vi "test.1dArrays.vi"(8 "error in":errorcluster, 10 "Data":variant, 11 "Command":string) -> (0 "error out":errorcluster, 3 "Return Data":variant)   [LabVIEW 2014]
uses:
  Private/Class/meth.Constructor.vi
  Private/Class/meth.Destructor.vi
  GLue.lvlib
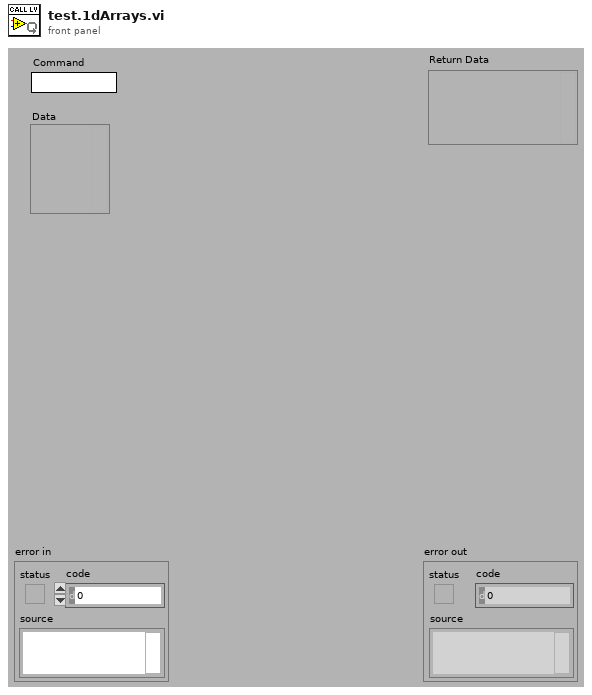
[diagram p1: front panel]
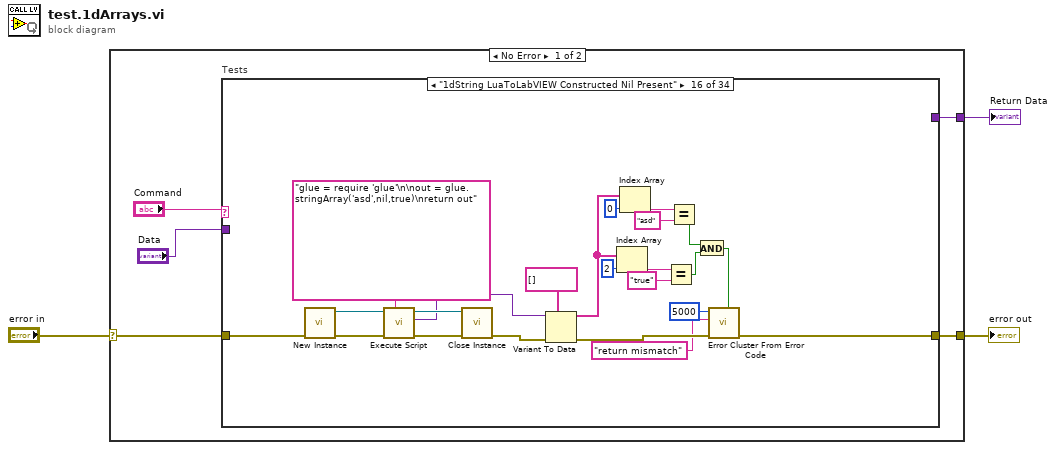
[diagram p0: block diagram]
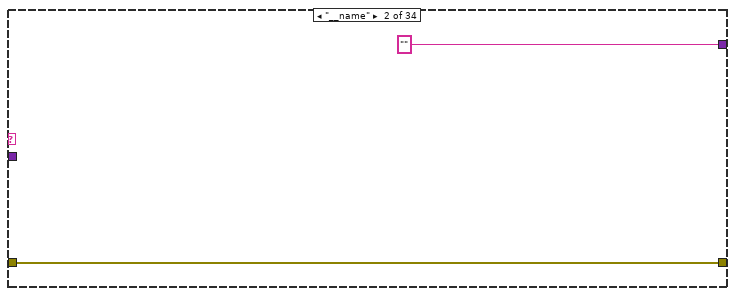
[diagram p3: hidden frame]
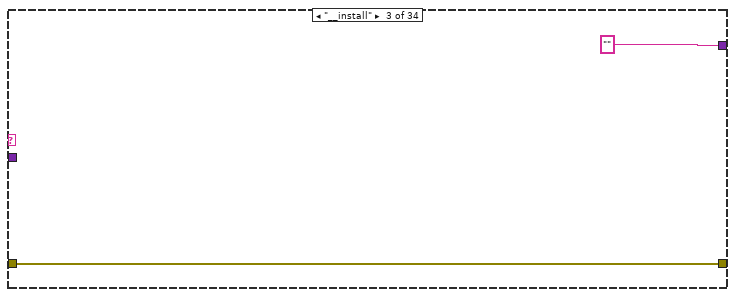
[diagram p4: hidden frame]
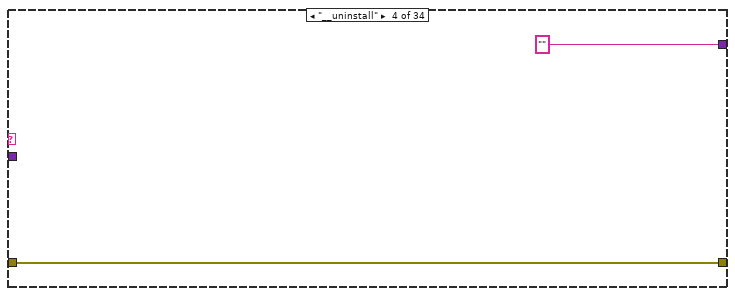
[diagram p5: hidden frame]
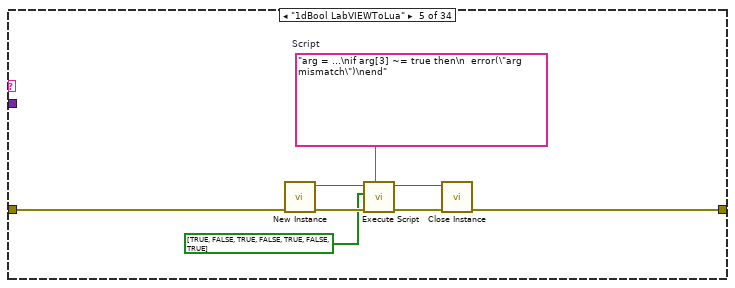
[diagram p6: hidden frame]
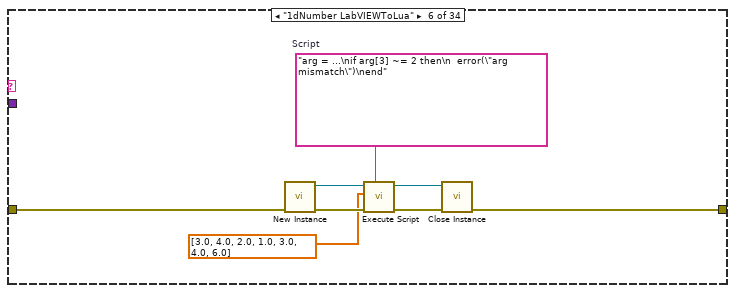
[diagram p7: hidden frame]
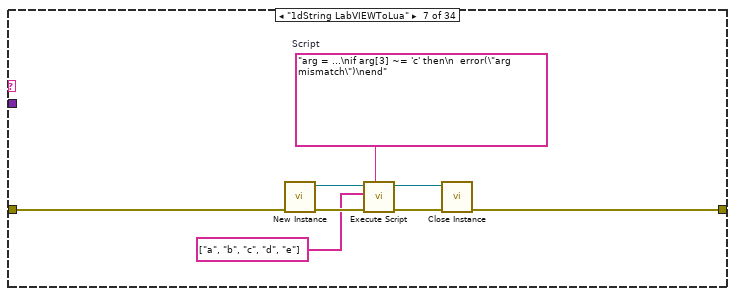
[diagram p8: hidden frame]
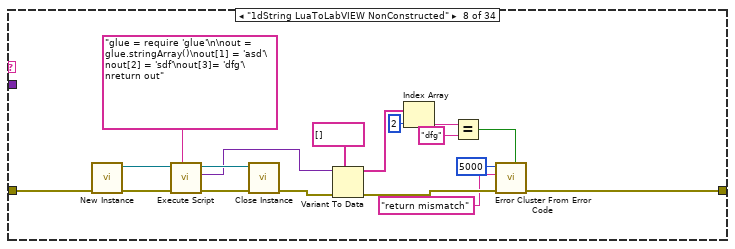
[diagram p9: hidden frame]
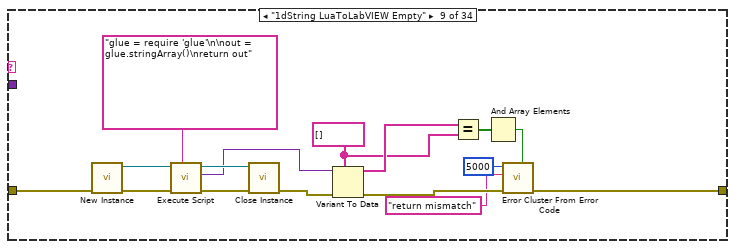
[diagram p10: hidden frame]
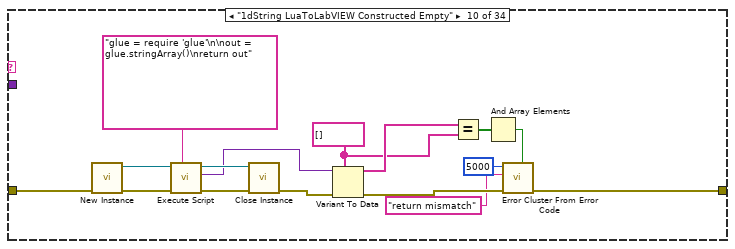
[diagram p11: hidden frame]
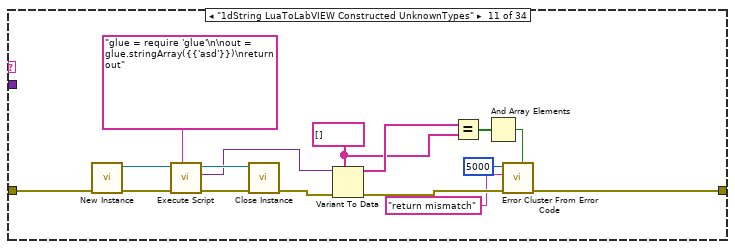
[diagram p12: hidden frame]
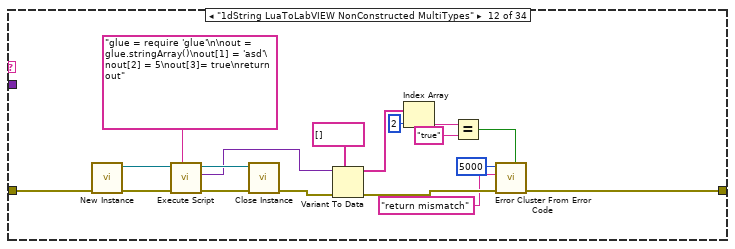
[diagram p13: hidden frame]
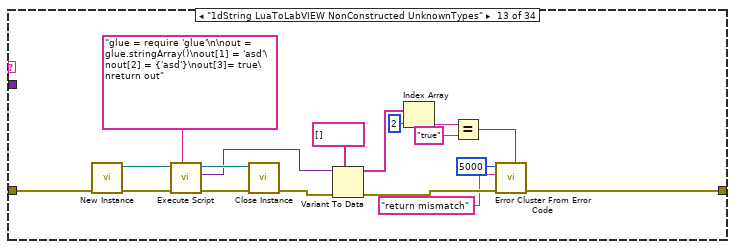
[diagram p14: hidden frame]
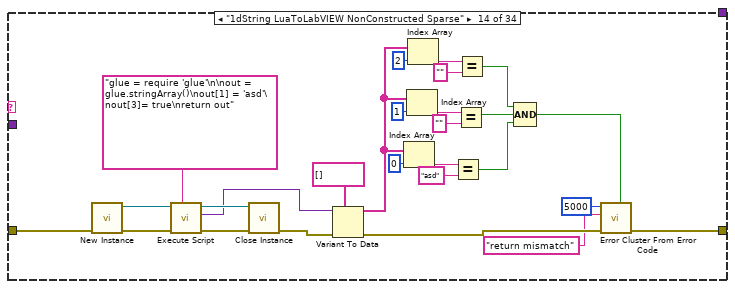
[diagram p15: hidden frame]
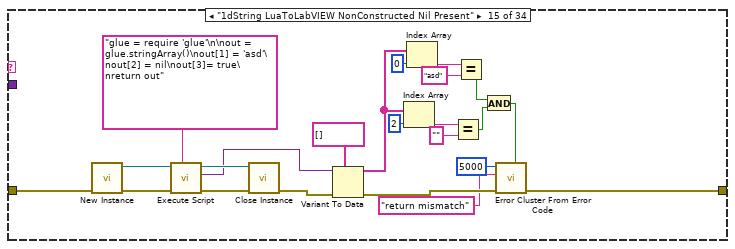
[diagram p16: hidden frame]
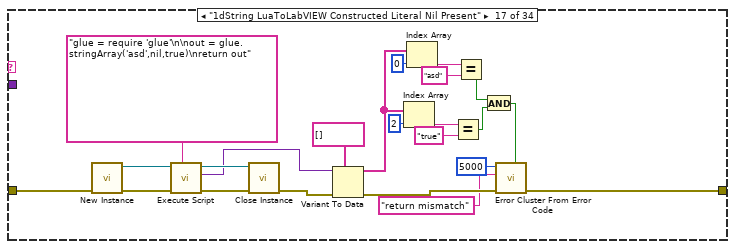
[diagram p17: hidden frame]
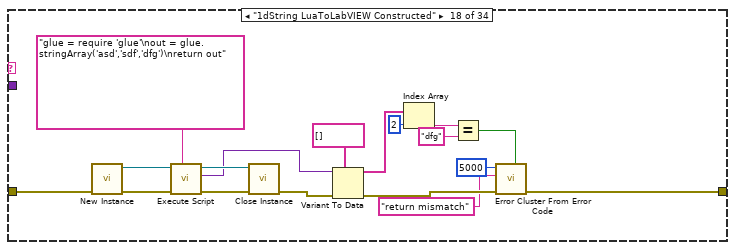
[diagram p18: hidden frame]
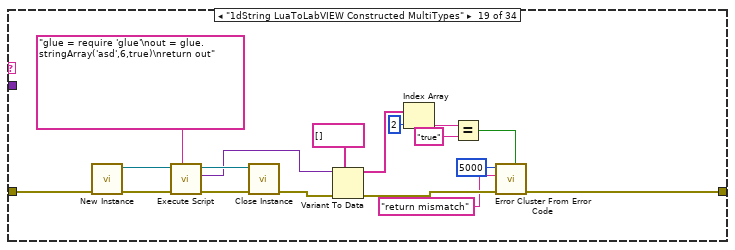
[diagram p19: hidden frame]
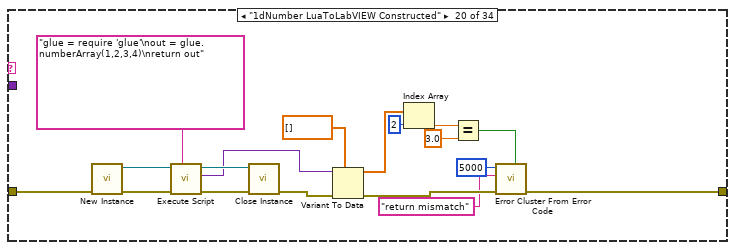
[diagram p20: hidden frame]
diagram:
  n1 = case shown="No Error" "error in" {
    selector: "error in" -> [w8 w579]
    tunnel: [w6 w579] -> w2
    tunnel: [w7 variant ("User Data")] -> w1
    frame No Error {
      n2 = case "Tests" shown="\"1dString LuaToLabVIEW Constructed Nil Present\"" "Command" {
        tunnel: w8 -> [w10 w11 w13 w15 w19 w27 w35 w53 w69 w85 w101 w119 w137 w164 w187 w210 w233 w251 w269 w287 w305 w321 w348 w375 w398 w420 w442 w459 w476 w494 w510 w526 w549 w572]
        tunnel: "Data" -> [w9 _ _ _ _ _ _ _ _ _ _ _ _ _ _ _ _ _ _ _ _ _ _ _ _ _ _ _ _ _ _ _ _ _]
        tunnel: [w9 "" "" "" _ _ _ _ _ _ _ _ _ _ _ _ _ _ _ _ _ _ _ _ _ _ _ _ _ _ _ _ _ _] -> w7
        tunnel: [w10 w11 w13 w15 w18 w26 w34 w48 w65 w81 w97 w114 w132 w159 w182 w205 w228 w246 w264 w283 w301 w317 w344 w371 w394 w416 w438 w455 w472 w490 w506 w522 w545 w568] -> w6
        frame Default {
        }
        frame "__name" {
        }
        frame "__install" {
        }
        frame "__uninstall" {
        }
        frame "1dBool LabVIEWToLua" {
          w24 = "arg = ...\nif arg[3] ~= true then\n  error(\"arg mismatch\")\nend"  # Script
          n3 = call "New Instance.vi"("error in"=w19) -> ("error out"=w20:errorcluster, "GLue out"=w21:refnum<class "class.GLue.lvclass">)  [unwired: 9 in]
          n4 = call "Execute Script.vi"("Script"=w24, "error in"=w20, "Argument Data"=bool[] [TRUE, FALSE, TRUE, FALSE, TRUE, FALSE, TRUE], "GLue in"=w21) -> ("error out"=w22:errorcluster, "GLue out"=w23:refnum<class "class.GLue.lvclass">)  [unwired: 5 in, 1 out]
          n5 = call "Close Instance.vi"("error in"=w22, "GLue in"=w23) -> ("error out"=w18:errorcluster)  [unwired: 9 in]
        }
        frame "1dNumber LabVIEWToLua" {
          w32 = "arg = ...\nif arg[3] ~= 2 then\n  error(\"arg mismatch\")\nend"  # Script
          n6 = call "New Instance.vi"("error in"=w27) -> ("error out"=w28:errorcluster, "GLue out"=w29:refnum<class "class.GLue.lvclass">)  [unwired: 9 in]
          n7 = call "Execute Script.vi"("Script"=w32, "error in"=w28, "Argument Data"=dbl[] [3.0, 4.0, 2.0, 1.0, 3.0, 4.0, 6.0], "GLue in"=w29) -> ("error out"=w30:errorcluster, "GLue out"=w31:refnum<class "class.GLue.lvclass">)  [unwired: 5 in, 1 out]
          n8 = call "Close Instance.vi"("error in"=w30, "GLue in"=w31) -> ("error out"=w26:errorcluster)  [unwired: 9 in]
        }
        frame "1dString LabVIEWToLua" {
          w40 = "arg = ...\nif arg[3] ~= 'c' then\n  error(\"arg mismatch\")\nend"  # Script
          n9 = call "New Instance.vi"("error in"=w35) -> ("error out"=w36:errorcluster, "GLue out"=w37:refnum<class "class.GLue.lvclass">)  [unwired: 9 in]
          n10 = call "Execute Script.vi"("Script"=w40, "error in"=w36, "Argument Data"=string[] ["a", "b", "c", "d", "e"], "GLue in"=w37) -> ("error out"=w38:errorcluster, "GLue out"=w39:refnum<class "class.GLue.lvclass">)  [unwired: 5 in, 1 out]
          n11 = call "Close Instance.vi"("error in"=w38, "GLue in"=w39) -> ("error out"=w34:errorcluster)  [unwired: 9 in]
        }
        frame "1dString LuaToLabVIEW NonConstructed" {
          n12 = call "New Instance.vi"("error in"=w53) -> ("error out"=w54:errorcluster, "GLue out"=w55:refnum<class "class.GLue.lvclass">)  [unwired: 9 in]
          n13 = call "Execute Script.vi"("Script"="glue = require 'glue'\n\nout = glue.stringArray()\nout[1] = 'asd'\nout[2] = 'sdf'\nout[3]= 'dfg'\nreturn out", "error in"=w54, "GLue in"=w55) -> ("error out"=w56:errorcluster, "Return Data"=w51:variant, "GLue out"=w57:refnum<class "class.GLue.lvclass">)  [unwired: 6 in]
          n14 = call "Close Instance.vi"("error in"=w56, "GLue in"=w57) -> ("error out"=w52:errorcluster)  [unwired: 9 in]
          n15 = Variant To Data(error in=w52, type=string[] [], Variant=w51) -> (data=w47:string[], error out=w49:errorcluster)
          n16 = Index Array(array=w47, index=2) -> (element=w45:string)
          n17 = Equal?(x=w45, y="dfg") -> (x = y?=w43:bool)
          n18 = call <vilib>:"Error Cluster From Error Code.vi"("is warning? (False)"=w43, "error in (no error)"=w49, "error message (\"\")"="return mismatch" ("error message (\"\")"), "error code (0)"=5000) -> ("error out"=w48:errorcluster)  [unwired: 5 in]
        }
        frame "1dString LuaToLabVIEW Empty" {
          w61 = string[] []
          n19 = call "New Instance.vi"("error in"=w69) -> ("error out"=w70:errorcluster, "GLue out"=w71:refnum<class "class.GLue.lvclass">)  [unwired: 9 in]
          n20 = call "Execute Script.vi"("Script"="glue = require 'glue'\n\nout = glue.stringArray()\nreturn out", "error in"=w70, "GLue in"=w71) -> ("error out"=w72:errorcluster, "Return Data"=w67:variant, "GLue out"=w73:refnum<class "class.GLue.lvclass">)  [unwired: 6 in]
          n21 = call "Close Instance.vi"("error in"=w72, "GLue in"=w73) -> ("error out"=w68:errorcluster)  [unwired: 9 in]
          n22 = Variant To Data(error in=w68, type=w61, Variant=w67) -> (data=w62:string[], error out=w66:errorcluster)
          n23 = Equal?(x=w62, y=w61) -> (x = y?=w60:bool[])
          n24 = And Array Elements(Boolean array=w60) -> (logical AND=w59:bool)
          n25 = call <vilib>:"Error Cluster From Error Code.vi"("is warning? (False)"=w59, "error in (no error)"=w66, "error message (\"\")"="return mismatch" ("error message (\"\")"), "error code (0)"=5000) -> ("error out"=w65:errorcluster)  [unwired: 5 in]
        }
        frame "1dString LuaToLabVIEW Constructed Empty" {
          w77 = string[] []
          n26 = call "New Instance.vi"("error in"=w85) -> ("error out"=w86:errorcluster, "GLue out"=w87:refnum<class "class.GLue.lvclass">)  [unwired: 9 in]
          n27 = call "Execute Script.vi"("Script"="glue = require 'glue'\n\nout = glue.stringArray()\nreturn out", "error in"=w86, "GLue in"=w87) -> ("error out"=w88:errorcluster, "Return Data"=w83:variant, "GLue out"=w89:refnum<class "class.GLue.lvclass">)  [unwired: 6 in]
          n28 = call "Close Instance.vi"("error in"=w88, "GLue in"=w89) -> ("error out"=w84:errorcluster)  [unwired: 9 in]
          n29 = Variant To Data(error in=w84, type=w77, Variant=w83) -> (data=w78:string[], error out=w82:errorcluster)
          n30 = Equal?(x=w78, y=w77) -> (x = y?=w76:bool[])
          n31 = And Array Elements(Boolean array=w76) -> (logical AND=w75:bool)
          n32 = call <vilib>:"Error Cluster From Error Code.vi"("is warning? (False)"=w75, "error in (no error)"=w82, "error message (\"\")"="return mismatch" ("error message (\"\")"), "error code (0)"=5000) -> ("error out"=w81:errorcluster)  [unwired: 5 in]
        }
        frame "1dString LuaToLabVIEW Constructed UnknownTypes" {
          w93 = string[] []
          n33 = call "New Instance.vi"("error in"=w101) -> ("error out"=w102:errorcluster, "GLue out"=w103:refnum<class "class.GLue.lvclass">)  [unwired: 9 in]
          n34 = call "Execute Script.vi"("Script"="glue = require 'glue'\n\nout = glue.stringArray({{'asd'}})\nreturn out", "error in"=w102, "GLue in"=w103) -> ("error out"=w104:errorcluster, "Return Data"=w99:variant, "GLue out"=w105:refnum<class "class.GLue.lvclass">)  [unwired: 6 in]
          n35 = call "Close Instance.vi"("error in"=w104, "GLue in"=w105) -> ("error out"=w100:errorcluster)  [unwired: 9 in]
          n36 = Variant To Data(error in=w100, type=w93, Variant=w99) -> (data=w94:string[], error out=w98:errorcluster)
          n37 = Equal?(x=w94, y=w93) -> (x = y?=w92:bool[])
          n38 = And Array Elements(Boolean array=w92) -> (logical AND=w91:bool)
          n39 = call <vilib>:"Error Cluster From Error Code.vi"("is warning? (False)"=w91, "error in (no error)"=w98, "error message (\"\")"="return mismatch" ("error message (\"\")"), "error code (0)"=5000) -> ("error out"=w97:errorcluster)  [unwired: 5 in]
        }
        frame "1dString LuaToLabVIEW NonConstructed MultiTypes" {
          n40 = call "New Instance.vi"("error in"=w119) -> ("error out"=w120:errorcluster, "GLue out"=w121:refnum<class "class.GLue.lvclass">)  [unwired: 9 in]
          n41 = call "Execute Script.vi"("Script"="glue = require 'glue'\n\nout = glue.stringArray()\nout[1] = 'asd'\nout[2] = 5\nout[3]= true\nreturn out", "error in"=w120, "GLue in"=w121) -> ("error out"=w122:errorcluster, "Return Data"=w117:variant, "GLue out"=w123:refnum<class "class.GLue.lvclass">)  [unwired: 6 in]
          n42 = call "Close Instance.vi"("error in"=w122, "GLue in"=w123) -> ("error out"=w118:errorcluster)  [unwired: 9 in]
          n43 = Variant To Data(error in=w118, type=string[] [], Variant=w117) -> (data=w113:string[], error out=w115:errorcluster)
          n44 = Index Array(array=w113, index=2) -> (element=w111:string)
          n45 = Equal?(x=w111, y="true") -> (x = y?=w109:bool)
          n46 = call <vilib>:"Error Cluster From Error Code.vi"("is warning? (False)"=w109, "error in (no error)"=w115, "error message (\"\")"="return mismatch" ("error message (\"\")"), "error code (0)"=5000) -> ("error out"=w114:errorcluster)  [unwired: 5 in]
        }
        frame "1dString LuaToLabVIEW NonConstructed UnknownTypes" {
          n47 = call "New Instance.vi"("error in"=w137) -> ("error out"=w138:errorcluster, "GLue out"=w139:refnum<class "class.GLue.lvclass">)  [unwired: 9 in]
          n48 = call "Execute Script.vi"("Script"="glue = require 'glue'\n\nout = glue.stringArray()\nout[1] = 'asd'\nout[2] = {'asd'}\nout[3]= true\nreturn out", "error in"=w138, "GLue in"=w139) -> ("error out"=w140:errorcluster, "Return Data"=w135:variant, "GLue out"=w141:refnum<class "class.GLue.lvclass">)  [unwired: 6 in]
          n49 = call "Close Instance.vi"("error in"=w140, "GLue in"=w141) -> ("error out"=w136:errorcluster)  [unwired: 9 in]
          n50 = Variant To Data(error in=w136, type=string[] [], Variant=w135) -> (data=w131:string[], error out=w133:errorcluster)
          n51 = Index Array(array=w131, index=2) -> (element=w129:string)
          n52 = Equal?(x=w129, y="true") -> (x = y?=w127:bool)
          n53 = call <vilib>:"Error Cluster From Error Code.vi"("is warning? (False)"=w127, "error in (no error)"=w133, "error message (\"\")"="return mismatch" ("error message (\"\")"), "error code (0)"=5000) -> ("error out"=w132:errorcluster)  [unwired: 5 in]
        }
        frame "1dString LuaToLabVIEW NonConstructed Sparse" {
          n54 = call "New Instance.vi"("error in"=w164) -> ("error out"=w165:errorcluster, "GLue out"=w166:refnum<class "class.GLue.lvclass">)  [unwired: 9 in]
          n55 = call "Execute Script.vi"("Script"="glue = require 'glue'\n\nout = glue.stringArray()\nout[1] = 'asd'\nout[3]= true\nreturn out", "error in"=w165, "GLue in"=w166) -> ("error out"=w167:errorcluster, "Return Data"=w162:variant, "GLue out"=w168:refnum<class "class.GLue.lvclass">)  [unwired: 6 in]
          n56 = call "Close Instance.vi"("error in"=w167, "GLue in"=w168) -> ("error out"=w163:errorcluster)  [unwired: 9 in]
          n57 = Variant To Data(error in=w163, type=string[] [], Variant=w162) -> (data=w147:string[], error out=w160:errorcluster)
          n58 = Index Array(array=w147, index=0) -> (element=w157:string)
          n59 = Index Array(array=w147, index=1) -> (element=w152:string)
          n60 = Index Array(array=w147, index=2) -> (element=w149:string)
          n61 = Equal?(x=w157, y="asd") -> (x = y?=w144:bool)
          n62 = Equal?(x=w152, y="") -> (x = y?=w145:bool)
          n63 = Equal?(x=w149, y="") -> (x = y?=w146:bool)
          n64 = Compound Arithmetic op=AND(w146, w145, w144) -> (w143:bool)
          n65 = call <vilib>:"Error Cluster From Error Code.vi"("is warning? (False)"=w143, "error in (no error)"=w160, "error message (\"\")"="return mismatch" ("error message (\"\")"), "error code (0)"=5000) -> ("error out"=w159:errorcluster)  [unwired: 5 in]
        }
        frame "1dString LuaToLabVIEW NonConstructed Nil Present" {
          n66 = call "New Instance.vi"("error in"=w187) -> ("error out"=w188:errorcluster, "GLue out"=w189:refnum<class "class.GLue.lvclass">)  [unwired: 9 in]
          n67 = call "Execute Script.vi"("Script"="glue = require 'glue'\n\nout = glue.stringArray()\nout[1] = 'asd'\nout[2] = nil\nout[3]= true\nreturn out", "error in"=w188, "GLue in"=w189) -> ("error out"=w190:errorcluster, "Return Data"=w185:variant, "GLue out"=w191:refnum<class "class.GLue.lvclass">)  [unwired: 6 in]
          n68 = call "Close Instance.vi"("error in"=w190, "GLue in"=w191) -> ("error out"=w186:errorcluster)  [unwired: 9 in]
          n69 = Variant To Data(error in=w186, type=string[] [], Variant=w185) -> (data=w173:string[], error out=w183:errorcluster)
          n70 = Index Array(array=w173, index=2) -> (element=w180:string)
          n71 = Index Array(array=w173, index=0) -> (element=w175:string)
          n72 = Equal?(x=w180, y="") -> (x = y?=w171:bool)
          n73 = Equal?(x=w175, y="asd") -> (x = y?=w172:bool)
          n74 = And(x=w172, y=w171) -> (x .and. y?=w170:bool)
          n75 = call <vilib>:"Error Cluster From Error Code.vi"("is warning? (False)"=w170, "error in (no error)"=w183, "error message (\"\")"="return mismatch" ("error message (\"\")"), "error code (0)"=5000) -> ("error out"=w182:errorcluster)  [unwired: 5 in]
        }
        frame "1dString LuaToLabVIEW Constructed Nil Present" {
          n76 = call "New Instance.vi"("error in"=w210) -> ("error out"=w211:errorcluster, "GLue out"=w212:refnum<class "class.GLue.lvclass">)  [unwired: 9 in]
          n77 = call "Execute Script.vi"("Script"="glue = require 'glue'\n\nout = glue.stringArray('asd',nil,true)\nreturn out", "error in"=w211, "GLue in"=w212) -> ("error out"=w213:errorcluster, "Return Data"=w208:variant, "GLue out"=w214:refnum<class "class.GLue.lvclass">)  [unwired: 6 in]
          n78 = call "Close Instance.vi"("error in"=w213, "GLue in"=w214) -> ("error out"=w209:errorcluster)  [unwired: 9 in]
          n79 = Variant To Data(error in=w209, type=string[] [], Variant=w208) -> (data=w197:string[], error out=w206:errorcluster)
          n80 = Index Array(array=w197, index=2) -> (element=w203:string)
          n81 = Index Array(array=w197, index=0) -> (element=w199:string)
          n82 = Equal?(x=w203, y="true") -> (x = y?=w195:bool)
          n83 = Equal?(x=w199, y="asd") -> (x = y?=w196:bool)
          n84 = And(x=w196, y=w195) -> (x .and. y?=w194:bool)
          n85 = call <vilib>:"Error Cluster From Error Code.vi"("is warning? (False)"=w194, "error in (no error)"=w206, "error message (\"\")"="return mismatch" ("error message (\"\")"), "error code (0)"=5000) -> ("error out"=w205:errorcluster)  [unwired: 5 in]
        }
        frame "1dString LuaToLabVIEW Constructed Literal Nil Present" {
          n86 = call "New Instance.vi"("error in"=w233) -> ("error out"=w234:errorcluster, "GLue out"=w235:refnum<class "class.GLue.lvclass">)  [unwired: 9 in]
          n87 = call "Execute Script.vi"("Script"="glue = require 'glue'\n\nout = glue.stringArray('asd',nil,true)\nreturn out", "error in"=w234, "GLue in"=w235) -> ("error out"=w236:errorcluster, "Return Data"=w231:variant, "GLue out"=w237:refnum<class "class.GLue.lvclass">)  [unwired: 6 in]
          n88 = call "Close Instance.vi"("error in"=w236, "GLue in"=w237) -> ("error out"=w232:errorcluster)  [unwired: 9 in]
          n89 = Variant To Data(error in=w232, type=string[] [], Variant=w231) -> (data=w219:string[], error out=w229:errorcluster)
          n90 = Index Array(array=w219, index=2) -> (element=w226:string)
          n91 = Index Array(array=w219, index=0) -> (element=w221:string)
          n92 = Equal?(x=w226, y="true") -> (x = y?=w217:bool)
          n93 = Equal?(x=w221, y="asd") -> (x = y?=w218:bool)
          n94 = And(x=w218, y=w217) -> (x .and. y?=w216:bool)
          n95 = call <vilib>:"Error Cluster From Error Code.vi"("is warning? (False)"=w216, "error in (no error)"=w229, "error message (\"\")"="return mismatch" ("error message (\"\")"), "error code (0)"=5000) -> ("error out"=w228:errorcluster)  [unwired: 5 in]
        }
        frame "1dString LuaToLabVIEW Constructed" {
          n96 = call "New Instance.vi"("error in"=w251) -> ("error out"=w252:errorcluster, "GLue out"=w253:refnum<class "class.GLue.lvclass">)  [unwired: 9 in]
          n97 = call "Execute Script.vi"("Script"="glue = require 'glue'\nout = glue.stringArray('asd','sdf','dfg')\nreturn out", "error in"=w252, "GLue in"=w253) -> ("error out"=w254:errorcluster, "Return Data"=w249:variant, "GLue out"=w255:refnum<class "class.GLue.lvclass">)  [unwired: 6 in]
          n98 = call "Close Instance.vi"("error in"=w254, "GLue in"=w255) -> ("error out"=w250:errorcluster)  [unwired: 9 in]
          n99 = Variant To Data(error in=w250, type=string[] [], Variant=w249) -> (data=w245:string[], error out=w247:errorcluster)
          n100 = Index Array(array=w245, index=2) -> (element=w243:string)
          n101 = Equal?(x=w243, y="dfg") -> (x = y?=w241:bool)
          n102 = call <vilib>:"Error Cluster From Error Code.vi"("is warning? (False)"=w241, "error in (no error)"=w247, "error message (\"\")"="return mismatch" ("error message (\"\")"), "error code (0)"=5000) -> ("error out"=w246:errorcluster)  [unwired: 5 in]
        }
        frame "1dString LuaToLabVIEW Constructed MultiTypes" {
          n103 = call "New Instance.vi"("error in"=w269) -> ("error out"=w270:errorcluster, "GLue out"=w271:refnum<class "class.GLue.lvclass">)  [unwired: 9 in]
          n104 = call "Execute Script.vi"("Script"="glue = require 'glue'\nout = glue.stringArray('asd',6,true)\nreturn out", "error in"=w270, "GLue in"=w271) -> ("error out"=w272:errorcluster, "Return Data"=w267:variant, "GLue out"=w273:refnum<class "class.GLue.lvclass">)  [unwired: 6 in]
          n105 = call "Close Instance.vi"("error in"=w272, "GLue in"=w273) -> ("error out"=w268:errorcluster)  [unwired: 9 in]
          n106 = Variant To Data(error in=w268, type=string[] [], Variant=w267) -> (data=w263:string[], error out=w265:errorcluster)
          n107 = Index Array(array=w263, index=2) -> (element=w261:string)
          n108 = Equal?(x=w261, y="true") -> (x = y?=w259:bool)
          n109 = call <vilib>:"Error Cluster From Error Code.vi"("is warning? (False)"=w259, "error in (no error)"=w265, "error message (\"\")"="return mismatch" ("error message (\"\")"), "error code (0)"=5000) -> ("error out"=w264:errorcluster)  [unwired: 5 in]
        }
        frame "1dNumber LuaToLabVIEW Constructed" {
          n110 = call "New Instance.vi"("error in"=w287) -> ("error out"=w288:errorcluster, "GLue out"=w289:refnum<class "class.GLue.lvclass">)  [unwired: 9 in]
          n111 = call "Execute Script.vi"("Script"="glue = require 'glue'\nout = glue.numberArray(1,2,3,4)\nreturn out", "error in"=w288, "GLue in"=w289) -> ("error out"=w290:errorcluster, "Return Data"=w285:variant, "GLue out"=w291:refnum<class "class.GLue.lvclass">)  [unwired: 6 in]
          n112 = call "Close Instance.vi"("error in"=w290, "GLue in"=w291) -> ("error out"=w286:errorcluster)  [unwired: 9 in]
          n113 = Variant To Data(error in=w286, type=dbl[] [], Variant=w285) -> (data=w282:dbl[], error out=w284:errorcluster)
          n114 = Index Array(array=w282, index=2) -> (element=w280:dbl)
          n115 = Equal?(x=w280, y=3.0) -> (x = y?=w279:bool)
          n116 = call <vilib>:"Error Cluster From Error Code.vi"("is warning? (False)"=w279, "error in (no error)"=w284, "error message (\"\")"="return mismatch" ("error message (\"\")"), "error code (0)"=5000) -> ("error out"=w283:errorcluster)  [unwired: 5 in]
        }
        frame "1dNumber LuaToLabVIEW Constructed Nil Present" {
          n117 = call "New Instance.vi"("error in"=w305) -> ("error out"=w306:errorcluster, "GLue out"=w307:refnum<class "class.GLue.lvclass">)  [unwired: 9 in]
          n118 = call "Execute Script.vi"("Script"="glue = require 'glue'\nout = glue.numberArray(1,2,nil,4)\nreturn out", "error in"=w306, "GLue in"=w307) -> ("error out"=w308:errorcluster, "Return Data"=w303:variant, "GLue out"=w309:refnum<class "class.GLue.lvclass">)  [unwired: 6 in]
          n119 = call "Close Instance.vi"("error in"=w308, "GLue in"=w309) -> ("error out"=w304:errorcluster)  [unwired: 9 in]
          n120 = Variant To Data(error in=w304, type=dbl[] [], Variant=w303) -> (data=w300:dbl[], error out=w302:errorcluster)
          n121 = Index Array(array=w300, index=1) -> (element=w298:dbl)
          n122 = Equal?(x=w298, y=2.0) -> (x = y?=w297:bool)
          n123 = call <vilib>:"Error Cluster From Error Code.vi"("is warning? (False)"=w297, "error in (no error)"=w302, "error message (\"\")"="return mismatch" ("error message (\"\")"), "error code (0)"=5000) -> ("error out"=w301:errorcluster)  [unwired: 5 in]
        }
        frame "1dNumber LuaToLabVIEW Constructed Empty" {
          w313 = dbl[] []
          n124 = call "New Instance.vi"("error in"=w321) -> ("error out"=w322:errorcluster, "GLue out"=w323:refnum<class "class.GLue.lvclass">)  [unwired: 9 in]
          n125 = call "Execute Script.vi"("Script"="glue = require 'glue'\nout = glue.numberArray()\nreturn out", "error in"=w322, "GLue in"=w323) -> ("error out"=w324:errorcluster, "Return Data"=w319:variant, "GLue out"=w325:refnum<class "class.GLue.lvclass">)  [unwired: 6 in]
          n126 = call "Close Instance.vi"("error in"=w324, "GLue in"=w325) -> ("error out"=w320:errorcluster)  [unwired: 9 in]
          n127 = Variant To Data(error in=w320, type=w313, Variant=w319) -> (data=w314:dbl[], error out=w318:errorcluster)
          n128 = Equal?(x=w314, y=w313) -> (x = y?=w312:bool[])
          n129 = And Array Elements(Boolean array=w312) -> (logical AND=w311:bool)
          n130 = call <vilib>:"Error Cluster From Error Code.vi"("is warning? (False)"=w311, "error in (no error)"=w318, "error message (\"\")"="return mismatch" ("error message (\"\")"), "error code (0)"=5000) -> ("error out"=w317:errorcluster)  [unwired: 5 in]
        }
        frame "1dNumber LuaToLabVIEW Constructed MultiTypes" {
          n131 = call "New Instance.vi"("error in"=w348) -> ("error out"=w349:errorcluster, "GLue out"=w350:refnum<class "class.GLue.lvclass">)  [unwired: 9 in]
          n132 = call "Execute Script.vi"("Script"="glue = require 'glue'\nout = glue.numberArray(1,'asd',true,4)\nreturn out", "error in"=w349, "GLue in"=w350) -> ("error out"=w351:errorcluster, "Return Data"=w346:variant, "GLue out"=w352:refnum<class "class.GLue.lvclass">)  [unwired: 6 in]
          n133 = call "Close Instance.vi"("error in"=w351, "GLue in"=w352) -> ("error out"=w347:errorcluster)  [unwired: 9 in]
          n134 = Variant To Data(error in=w347, type=dbl[] [], Variant=w346) -> (data=w328:dbl[], error out=w345:errorcluster)
          n135 = Index Array(array=w328, index=0) -> (element=w342:dbl)
          n136 = Index Array(array=w328, index=3) -> (element=w336:dbl)
          n137 = Index Array(array=w328, index=1) -> (element=w330:dbl)
          n138 = Equal?(x=w342, y=1.0) -> (x = y?=w333:bool)
          n139 = Equal?(x=w336, y=4.0) -> (x = y?=w334:bool)
          n140 = Equal?(x=w330, y=0.0) -> (x = y?=w327:bool)
          n141 = Compound Arithmetic op=AND(w327, w334, w333) -> (w332:bool)
          n142 = call <vilib>:"Error Cluster From Error Code.vi"("is warning? (False)"=w332, "error in (no error)"=w345, "error message (\"\")"="return mismatch" ("error message (\"\")"), "error code (0)"=5000) -> ("error out"=w344:errorcluster)  [unwired: 5 in]
        }
        frame "1dNumber LuaToLabVIEW NonConstructed MultiTypes" {
          n143 = call "New Instance.vi"("error in"=w375) -> ("error out"=w376:errorcluster, "GLue out"=w377:refnum<class "class.GLue.lvclass">)  [unwired: 9 in]
          n144 = call "Execute Script.vi"("Script"="glue = require 'glue'\nout = glue.numberArray()\nout[1] = 1\nout[2] = 'asd'\nout[3] = true\nout[4] = 2\nreturn out", "error in"=w376, "GLue in"=w377) -> ("error out"=w378:errorcluster, "Return Data"=w373:variant, "GLue out"=w379:refnum<class "class.GLue.lvclass">)  [unwired: 6 in]
          n145 = call "Close Instance.vi"("error in"=w378, "GLue in"=w379) -> ("error out"=w374:errorcluster)  [unwired: 9 in]
          n146 = Variant To Data(error in=w374, type=dbl[] [], Variant=w373) -> (data=w355:dbl[], error out=w372:errorcluster)
          n147 = Index Array(array=w355, index=0) -> (element=w369:dbl)
          n148 = Index Array(array=w355, index=3) -> (element=w363:dbl)
          n149 = Index Array(array=w355, index=1) -> (element=w357:dbl)
          n150 = Equal?(x=w369, y=1.0) -> (x = y?=w360:bool)
          n151 = Equal?(x=w363, y=2.0) -> (x = y?=w361:bool)
          n152 = Equal?(x=w357, y=0.0) -> (x = y?=w354:bool)
          n153 = Compound Arithmetic op=AND(w354, w361, w360) -> (w359:bool)
          n154 = call <vilib>:"Error Cluster From Error Code.vi"("is warning? (False)"=w359, "error in (no error)"=w372, "error message (\"\")"="return mismatch" ("error message (\"\")"), "error code (0)"=5000) -> ("error out"=w371:errorcluster)  [unwired: 5 in]
        }
        frame "1dBool LuaToLabVIEW NonConstructed" {
          n155 = call "New Instance.vi"("error in"=w398) -> ("error out"=w399:errorcluster, "GLue out"=w400:refnum<class "class.GLue.lvclass">)  [unwired: 9 in]
          n156 = call "Execute Script.vi"("Script"="glue = require 'glue'\nout = glue.boolArray()\nout[1] = false\nout[2] = true\nout[3] = true\nout[4] = false\nreturn out", "error in"=w399, "GLue in"=w400) -> ("error out"=w401:errorcluster, "Return Data"=w396:variant, "GLue out"=w402:refnum<class "class.GLue.lvclass">)  [unwired: 6 in]
          n157 = call "Close Instance.vi"("error in"=w401, "GLue in"=w402) -> ("error out"=w397:errorcluster)  [unwired: 9 in]
          n158 = Variant To Data(error in=w397, type=bool[] [], Variant=w396) -> (data=w386:bool[], error out=w395:errorcluster)
          n159 = Index Array(array=w386, index=0) -> (element=w385:bool)
          n160 = Index Array(array=w386, index=3) -> (element=w384:bool)
          n161 = Index Array(array=w386, index=1) -> (element=w383:bool)
          n162 = Not(x=w384) -> (.not. x?=w382:bool)
          n163 = Not(x=w385) -> (.not. x?=w381:bool)
          n164 = Compound Arithmetic op=AND(w383, w382, w381) -> (w388:bool)
          n165 = call <vilib>:"Error Cluster From Error Code.vi"("is warning? (False)"=w388, "error in (no error)"=w395, "error message (\"\")"="return mismatch" ("error message (\"\")"), "error code (0)"=5000) -> ("error out"=w394:errorcluster)  [unwired: 5 in]
        }
        frame "1dBool LuaToLabVIEW NonConstructed MultiTypes" {
          n166 = call "New Instance.vi"("error in"=w420) -> ("error out"=w421:errorcluster, "GLue out"=w422:refnum<class "class.GLue.lvclass">)  [unwired: 9 in]
          n167 = call "Execute Script.vi"("Script"="glue = require 'glue'\nout = glue.boolArray()\nout[1] = false\nout[2] = 5\nout[3] = 'false'\nreturn out", "error in"=w421, "GLue in"=w422) -> ("error out"=w423:errorcluster, "Return Data"=w418:variant, "GLue out"=w424:refnum<class "class.GLue.lvclass">)  [unwired: 6 in]
          n168 = call "Close Instance.vi"("error in"=w423, "GLue in"=w424) -> ("error out"=w419:errorcluster)  [unwired: 9 in]
          n169 = Variant To Data(error in=w419, type=bool[] [], Variant=w418) -> (data=w408:bool[], error out=w417:errorcluster)
          n170 = Index Array(array=w408, index=0) -> (element=w407:bool)
          n171 = Index Array(array=w408, index=1) -> (element=w404:bool)
          n172 = Index Array(array=w408, index=2) -> (element=w406:bool)
          n173 = Not(x=w407) -> (.not. x?=w405:bool)
          n174 = Compound Arithmetic op=AND(w406, w404, w405) -> (w410:bool)
          n175 = call <vilib>:"Error Cluster From Error Code.vi"("is warning? (False)"=w410, "error in (no error)"=w417, "error message (\"\")"="return mismatch" ("error message (\"\")"), "error code (0)"=5000) -> ("error out"=w416:errorcluster)  [unwired: 5 in]
        }
        frame "1dBool LuaToLabVIEW Constructed MultiTypes" {
          n176 = call "New Instance.vi"("error in"=w442) -> ("error out"=w443:errorcluster, "GLue out"=w444:refnum<class "class.GLue.lvclass">)  [unwired: 9 in]
          n177 = call "Execute Script.vi"("Script"="glue = require 'glue'\nout = glue.boolArray(false,5,'test')\nreturn out", "error in"=w443, "GLue in"=w444) -> ("error out"=w445:errorcluster, "Return Data"=w440:variant, "GLue out"=w446:refnum<class "class.GLue.lvclass">)  [unwired: 6 in]
          n178 = call "Close Instance.vi"("error in"=w445, "GLue in"=w446) -> ("error out"=w441:errorcluster)  [unwired: 9 in]
          n179 = Variant To Data(error in=w441, type=bool[] [], Variant=w440) -> (data=w430:bool[], error out=w439:errorcluster)
          n180 = Index Array(array=w430, index=0) -> (element=w429:bool)
          n181 = Index Array(array=w430, index=1) -> (element=w426:bool)
          n182 = Index Array(array=w430, index=2) -> (element=w428:bool)
          n183 = Not(x=w429) -> (.not. x?=w427:bool)
          n184 = Compound Arithmetic op=AND(w428, w426, w427) -> (w432:bool)
          n185 = call <vilib>:"Error Cluster From Error Code.vi"("is warning? (False)"=w432, "error in (no error)"=w439, "error message (\"\")"="return mismatch" ("error message (\"\")"), "error code (0)"=5000) -> ("error out"=w438:errorcluster)  [unwired: 5 in]
        }
        frame "1dBool LuaToLabVIEW NonConstructed Sparse" {
          n186 = call "New Instance.vi"("error in"=w459) -> ("error out"=w460:errorcluster, "GLue out"=w461:refnum<class "class.GLue.lvclass">)  [unwired: 9 in]
          n187 = call "Execute Script.vi"("Script"="glue = require 'glue'\nout = glue.boolArray()\nout[1] = true\nout[2] = nil\nout[3] = true\nreturn out", "error in"=w460, "GLue in"=w461) -> ("error out"=w462:errorcluster, "Return Data"=w457:variant, "GLue out"=w463:refnum<class "class.GLue.lvclass">)  [unwired: 6 in]
          n188 = call "Close Instance.vi"("error in"=w462, "GLue in"=w463) -> ("error out"=w458:errorcluster)  [unwired: 9 in]
          n189 = Variant To Data(error in=w458, type=bool[] [], Variant=w457) -> (data=w449:bool[], error out=w456:errorcluster)
          n190 = Index Array(array=w449, index=0) -> (element=w448:bool)
          n191 = Compound Arithmetic op=AND(w448) -> (w450:bool)
          n192 = call <vilib>:"Error Cluster From Error Code.vi"("is warning? (False)"=w450, "error in (no error)"=w456, "error message (\"\")"="return mismatch" ("error message (\"\")"), "error code (0)"=5000) -> ("error out"=w455:errorcluster)  [unwired: 5 in]
        }
        frame "1dBool LuaToLabVIEW Constructed Nil Present" {
          n193 = call "New Instance.vi"("error in"=w476) -> ("error out"=w477:errorcluster, "GLue out"=w478:refnum<class "class.GLue.lvclass">)  [unwired: 9 in]
          n194 = call "Execute Script.vi"("Script"="glue = require 'glue'\nout = glue.boolArray(true,nil,true)\nreturn out", "error in"=w477, "GLue in"=w478) -> ("error out"=w479:errorcluster, "Return Data"=w474:variant, "GLue out"=w480:refnum<class "class.GLue.lvclass">)  [unwired: 6 in]
          n195 = call "Close Instance.vi"("error in"=w479, "GLue in"=w480) -> ("error out"=w475:errorcluster)  [unwired: 9 in]
          n196 = Variant To Data(error in=w475, type=bool[] [], Variant=w474) -> (data=w466:bool[], error out=w473:errorcluster)
          n197 = Index Array(array=w466, index=0) -> (element=w465:bool)
          n198 = Compound Arithmetic op=AND(w465) -> (w467:bool)
          n199 = call <vilib>:"Error Cluster From Error Code.vi"("is warning? (False)"=w467, "error in (no error)"=w473, "error message (\"\")"="return mismatch" ("error message (\"\")"), "error code (0)"=5000) -> ("error out"=w472:errorcluster)  [unwired: 5 in]
        }
        frame "1dBool LuaToLabVIEW NonConstructed Nil Present" {
          n200 = call "New Instance.vi"("error in"=w494) -> ("error out"=w495:errorcluster, "GLue out"=w496:refnum<class "class.GLue.lvclass">)  [unwired: 9 in]
          n201 = call "Execute Script.vi"("Script"="glue = require 'glue'\nout = glue.boolArray()\nout[1] = false\nout[2] = nil\nout[3] = 'false'\nreturn out", "error in"=w495, "GLue in"=w496) -> ("error out"=w497:errorcluster, "Return Data"=w492:variant, "GLue out"=w498:refnum<class "class.GLue.lvclass">)  [unwired: 6 in]
          n202 = call "Close Instance.vi"("error in"=w497, "GLue in"=w498) -> ("error out"=w493:errorcluster)  [unwired: 9 in]
          n203 = Variant To Data(error in=w493, type=bool[] [], Variant=w492) -> (data=w484:bool[], error out=w491:errorcluster)
          n204 = Index Array(array=w484, index=0) -> (element=w483:bool)
          n205 = Not(x=w483) -> (.not. x?=w482:bool)
          n206 = Compound Arithmetic op=AND(w482) -> (w485:bool)
          n207 = call <vilib>:"Error Cluster From Error Code.vi"("is warning? (False)"=w485, "error in (no error)"=w491, "error message (\"\")"="return mismatch" ("error message (\"\")"), "error code (0)"=5000) -> ("error out"=w490:errorcluster)  [unwired: 5 in]
        }
        frame "1dBool LuaToLabVIEW NonConstructed Empty" {
          w502 = bool[] []
          n208 = call "New Instance.vi"("error in"=w510) -> ("error out"=w511:errorcluster, "GLue out"=w512:refnum<class "class.GLue.lvclass">)  [unwired: 9 in]
          n209 = call "Execute Script.vi"("Script"="glue = require 'glue'\nout = glue.boolArray()\nreturn out", "error in"=w511, "GLue in"=w512) -> ("error out"=w513:errorcluster, "Return Data"=w508:variant, "GLue out"=w514:refnum<class "class.GLue.lvclass">)  [unwired: 6 in]
          n210 = call "Close Instance.vi"("error in"=w513, "GLue in"=w514) -> ("error out"=w509:errorcluster)  [unwired: 9 in]
          n211 = Variant To Data(error in=w509, type=w502, Variant=w508) -> (data=w503:bool[], error out=w507:errorcluster)
          n212 = Equal?(x=w503, y=w502) -> (x = y?=w501:bool[])
          n213 = And Array Elements(Boolean array=w501) -> (logical AND=w500:bool)
          n214 = call <vilib>:"Error Cluster From Error Code.vi"("is warning? (False)"=w500, "error in (no error)"=w507, "error message (\"\")"="return mismatch" ("error message (\"\")"), "error code (0)"=5000) -> ("error out"=w506:errorcluster)  [unwired: 5 in]
        }
        frame "1dBool LuaToLabVIEW Constructed Empty" {
          w518 = bool[] []
          n215 = call "New Instance.vi"("error in"=w526) -> ("error out"=w527:errorcluster, "GLue out"=w528:refnum<class "class.GLue.lvclass">)  [unwired: 9 in]
          n216 = call "Execute Script.vi"("Script"="glue = require 'glue'\nout = glue.boolArray()\nreturn out", "error in"=w527, "GLue in"=w528) -> ("error out"=w529:errorcluster, "Return Data"=w524:variant, "GLue out"=w530:refnum<class "class.GLue.lvclass">)  [unwired: 6 in]
          n217 = call "Close Instance.vi"("error in"=w529, "GLue in"=w530) -> ("error out"=w525:errorcluster)  [unwired: 9 in]
          n218 = Variant To Data(error in=w525, type=w518, Variant=w524) -> (data=w519:bool[], error out=w523:errorcluster)
          n219 = Equal?(x=w519, y=w518) -> (x = y?=w517:bool[])
          n220 = And Array Elements(Boolean array=w517) -> (logical AND=w516:bool)
          n221 = call <vilib>:"Error Cluster From Error Code.vi"("is warning? (False)"=w516, "error in (no error)"=w523, "error message (\"\")"="return mismatch" ("error message (\"\")"), "error code (0)"=5000) -> ("error out"=w522:errorcluster)  [unwired: 5 in]
        }
        frame "1dNumber LuaToLabVIEW NonConstructed Sparse" {
          n222 = call "New Instance.vi"("error in"=w549) -> ("error out"=w550:errorcluster, "GLue out"=w551:refnum<class "class.GLue.lvclass">)  [unwired: 9 in]
          n223 = call "Execute Script.vi"("Script"="glue = require 'glue'\nout = glue.numberArray()\nout[1] = 1\nout[4] = 2\nreturn out", "error in"=w550, "GLue in"=w551) -> ("error out"=w552:errorcluster, "Return Data"=w547:variant, "GLue out"=w553:refnum<class "class.GLue.lvclass">)  [unwired: 6 in]
          n224 = call "Close Instance.vi"("error in"=w552, "GLue in"=w553) -> ("error out"=w548:errorcluster)  [unwired: 9 in]
          n225 = Variant To Data(error in=w548, type=dbl[] [], Variant=w547) -> (data=w532:dbl[], error out=w546:errorcluster)
          n226 = Index Array(array=w532, index=0) -> (element=w543:dbl)
          n227 = Index Array(array=w532, index=3) -> (element=w537:dbl)
          n228 = Equal?(x=w543, y=1.0) -> (x = y?=w534:bool)
          n229 = Equal?(x=w537, y=0.0) -> (x = y?=w535:bool)
          n230 = Compound Arithmetic op=AND(w535, w534) -> (w533:bool)
          n231 = call <vilib>:"Error Cluster From Error Code.vi"("is warning? (False)"=w533, "error in (no error)"=w546, "error message (\"\")"="return mismatch" ("error message (\"\")"), "error code (0)"=5000) -> ("error out"=w545:errorcluster)  [unwired: 5 in]
        }
        frame "1dNumber LuaToLabVIEW NonConstructed Nil Present" {
          n232 = call "New Instance.vi"("error in"=w572) -> ("error out"=w573:errorcluster, "GLue out"=w574:refnum<class "class.GLue.lvclass">)  [unwired: 9 in]
          n233 = call "Execute Script.vi"("Script"="glue = require 'glue'\nout = glue.numberArray()\nout[1] = 1\nout[2] = 'asd'\nout[3] = nil\nout[4] = 2\nreturn out", "error in"=w573, "GLue in"=w574) -> ("error out"=w575:errorcluster, "Return Data"=w570:variant, "GLue out"=w576:refnum<class "class.GLue.lvclass">)  [unwired: 6 in]
          n234 = call "Close Instance.vi"("error in"=w575, "GLue in"=w576) -> ("error out"=w571:errorcluster)  [unwired: 9 in]
          n235 = Variant To Data(error in=w571, type=dbl[] [], Variant=w570) -> (data=w557:dbl[], error out=w569:errorcluster)
          n236 = Index Array(array=w557, index=0) -> (element=w566:dbl)
          n237 = Index Array(array=w557, index=1) -> (element=w559:dbl)
          n238 = Equal?(x=w566, y=1.0) -> (x = y?=w555:bool)
          n239 = Equal?(x=w559, y=0.0) -> (x = y?=w556:bool)
          n240 = Compound Arithmetic op=AND(w556, w555) -> (w561:bool)
          n241 = call <vilib>:"Error Cluster From Error Code.vi"("is warning? (False)"=w561, "error in (no error)"=w569, "error message (\"\")"="return mismatch" ("error message (\"\")"), "error code (0)"=5000) -> ("error out"=w568:errorcluster)  [unwired: 5 in]
        }
      }
    }
    frame Error {
    }
  }
  "Return Data" <- w1
  "error out" <- w2
